vi "Definition Cluster.vi"(11 "ID in":refnum<class "ID.lvclass">) -> (2 "Definition":variant, 3 "ID out":refnum<class "ID.lvclass">)   [LabVIEW 2020, in "Conditum.lvlib" / "Columns.lvlib" / "ID.lvclass"]
uses:
  ID.lvclass
  ID.lvclass/ID.ctl
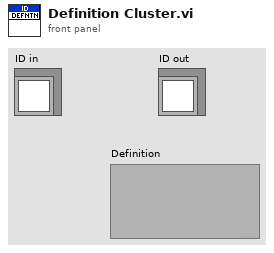
[diagram p1: front panel]
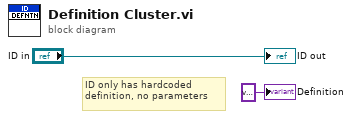
[diagram p0: block diagram]
diagram:
  # "ID only has hardcoded definition, no parameters"
  "ID out" <- "ID in"
  "Definition" <- variant ("Definition")
